vi "Get Random Free Point_v2.vi"(7 "Safe Area?":bool, 8 "error in (no error)":errorcluster, 11 "Board Game in":refnum<class "Board Game.lvclass">) -> (0 "error out":errorcluster, 3 "Position":cluster{"X":dbl, "Y":dbl})   [LabVIEW 2021, in "Board Game.lvclass"]
uses:
  Board Game.lvclass
  Board Game.lvclass/Board Game.ctl
  Snake_class/Snake.lvclass
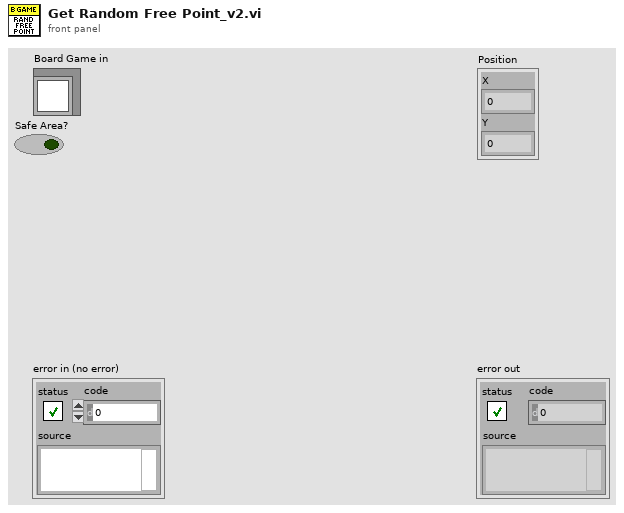
[diagram p1: front panel]
types:
  T1 = typedef "GameEl.lvclass/Enum Direction.ctl" = enum16{"Up", "Down", "Forward", "Backward"}
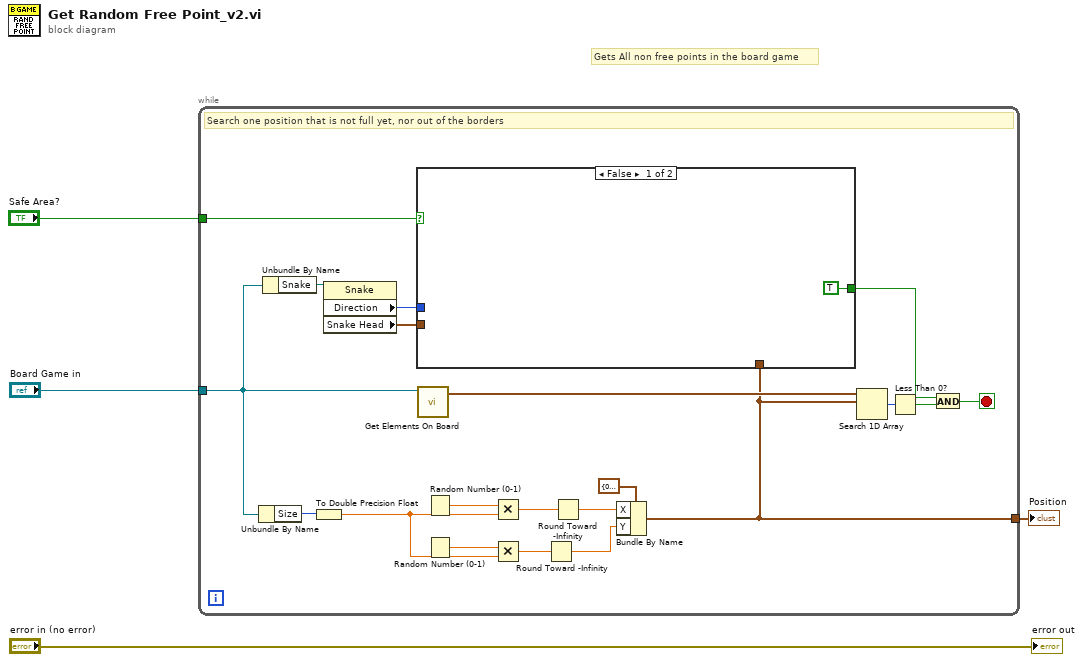
[diagram p0: block diagram]
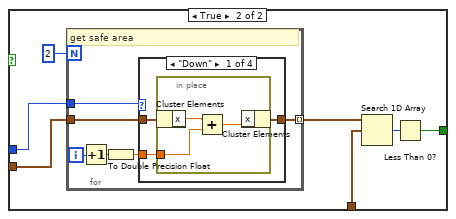
[diagram p2: hidden frame]
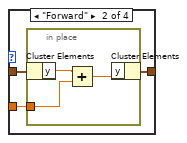
[diagram p3: hidden frame]
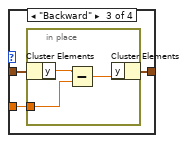
[diagram p4: hidden frame]
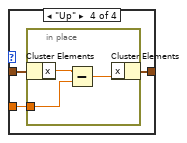
[diagram p5: hidden frame]
diagram:
  # "Gets All non free points in the board game"
  n1 = while {
    tunnel: "Board Game in" -> [w11]
    tunnel: [w7] -> w2
    tunnel: "Safe Area?" -> [w12]
    stop <- w6 stop-if-true
    # "Search one position that is not full yet, nor out of the borders"
    n2 = Unbundle By Name(w11) -> ("Size"=w13:u16)
    n3 = Unbundle By Name(w11) -> ("Snake"=w10:refnum<class "Snake.lvclass">)
    n4 = To Double Precision Float(number=w13) -> (double precision float=w17:dbl)
    n5 = property class="Snake"(reference=w10) -> ("Direction"=w8:T1, "Snake Head"=w9:cluster{"x":dbl, "y":dbl})  [unwired: 1 in, 2 out]
    n6 = call "Get Elements On Board.vi"("Board Game in"=w11) -> ("position"=w16:cluster{"x":dbl, "y":dbl}[])  [unwired: 9 in, 1 out]
    n7 = Random Number (0-1)() -> (number: 0 to 1=w24:dbl)
    n8 = Random Number (0-1)() -> (number: 0 to 1=w23:dbl)
    n9 = Multiply(x=w24, y=w17) -> (x*y=w21:dbl)
    n10 = Multiply(x=w23, y=w17) -> (x*y=w20:dbl)
    n11 = Round Toward -Infinity(1:w20) -> (0:w18:dbl)
    n12 = Round Toward -Infinity(1:w21) -> (0:w19:dbl)
    n13 = Bundle By Name(cluster=cluster{"X":dbl, "Y":dbl} {"X"=0.0, "Y"=0.0} ("Position"), "X"=w19, "Y"=w18) -> (w7:cluster{"X":dbl, "Y":dbl})
    n14 = case shown="False" w12 {
      tunnel: w9 -> [_ w31]
      tunnel: w8 -> [_ w30]
      tunnel: w7 -> [_ w27]
      tunnel: [TRUE w26] -> w5
      frame False {
      }
      frame True {
        n15 = for {
          N: 2 -> [_]
          tunnel: w30 -> [w37]
          tunnel: w31 -> [w36]
          tunnel: [w33] -> w28 mode=indexing
          i -> [w38]
          # "get safe area"
          n16 = Increment(x=w38) -> (x+1=w35:i32)
          n17 = To Double Precision Float(number=w35) -> (double precision float=w34:dbl)
          n18 = case shown="\"Down\"" w37 {
            tunnel: w36 -> [w41 w47 w53 w59]
            tunnel: w34 -> [w40 w46 w52 w58]
            tunnel: [w39 w45 w51 w57] -> w33
            frame "Down" {
              n19 = in-place {
                in-place-border: w40 -> [w43]
                n20 = in-place-cluster #1(w41) -> ("x"=w44:dbl)
                n21 = Add(x=w44, y=w43) -> (x+y=w42:dbl)
                n22 = in-place-cluster #1("x"=w42) -> (w39:cluster{"x":dbl, "y":dbl})
              }
            }
            frame "Forward" {
              n23 = in-place {
                in-place-border: w46 -> [w49]
                n24 = in-place-cluster #2(w47) -> ("y"=w50:dbl)
                n25 = Add(x=w50, y=w49) -> (x+y=w48:dbl)
                n26 = in-place-cluster #2("y"=w48) -> (w45:cluster{"x":dbl, "y":dbl})
              }
            }
            frame "Backward" {
              n27 = in-place {
                in-place-border: w52 -> [w55]
                n28 = in-place-cluster #3(w53) -> ("y"=w56:dbl)
                n29 = Subtract(x=w56, y=w55) -> (x-y=w54:dbl)
                n30 = in-place-cluster #3("y"=w54) -> (w51:cluster{"x":dbl, "y":dbl})
              }
            }
            frame "Up" {
              n31 = in-place {
                in-place-border: w58 -> [w61]
                n32 = in-place-cluster #4(w59) -> ("x"=w62:dbl)
                n33 = Subtract(x=w62, y=w61) -> (x-y=w60:dbl)
                n34 = in-place-cluster #4("x"=w60) -> (w57:cluster{"x":dbl, "y":dbl})
              }
            }
          }
        }
        n35 = Search 1D Array(1D array=w28, element=w27) -> (index of element=w29:i32)  [unwired: 1 in]
        n36 = Less Than 0?(x=w29) -> (x < 0?=w26:bool)
      }
    }
    n37 = Search 1D Array(1D array=w16, element=w7) -> (index of element=w15:i32)  [unwired: 1 in]
    n38 = Less Than 0?(x=w15) -> (x < 0?=w14:bool)
    n39 = And(x=w5, y=w14) -> (x .and. y?=w6:bool)
  }
  "Position" <- w2
  "error out" <- "error in (no error)"
